vi "Project - Symbols.vi"(7 "Msg Chain":string, 8 "error in (no error)":errorcluster {"code" format="Error %.0f"}, 10 "Project Doc":refnum<class "Project Documentation.lvclass">, 11 "VIDoc Printer - Confluence In":refnum<class "VIDoc Printer - Confluence.lvclass">) -> (0 "error out":errorcluster {"code" format="Error %.0f"}, 3 "VIDoc Printer - Confluence Out":refnum<class "VIDoc Printer - Confluence.lvclass">)   [LabVIEW 2023, in "VIDoc Printer - Confluence.lvlib" / "VIDoc Printer - Confluence.lvclass"]
uses:
  VIDoc Printer - Confluence.lvclass
  Parsing/Project Documentation/Project Documentation.lvclass
  Confluence Formatting/Types/Format Combo Box.ctl
  Parsing/Project Documentation/Project Documentation.lvclass/Project Documentation.ctl
  Parsing/Project Documentation/Get Conditional Disable Symbols.vi
  <userlib>/_PetranWay/LabVIEW Confluence API/Source/Confluence/HTML/Create Table (Responsive).vi
  VIDoc Printer - Confluence.lvclass/VIDoc Printer - Confluence.ctl
  <userlib>/_PetranWay/LabVIEW Confluence API/Source/PetranWay_Confluence API.lvlib
  Confluence Formatting/Confluence Formatting.lvlib
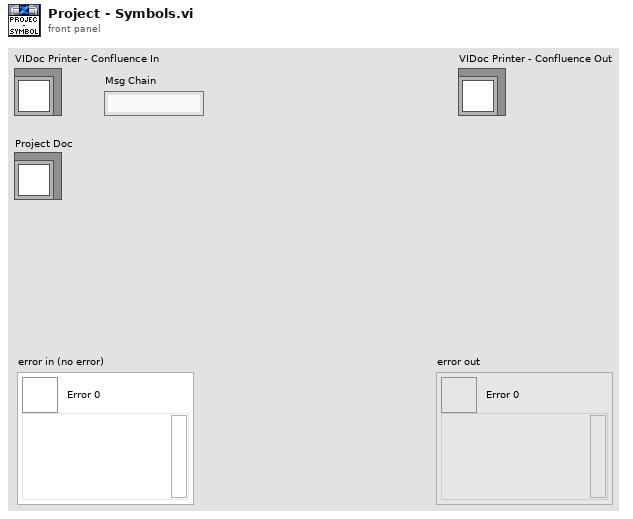
[diagram p1: front panel]
types:
  T1 = typedef "Confluence Formatting.lvlib/Format Combo Box.ctl" = string
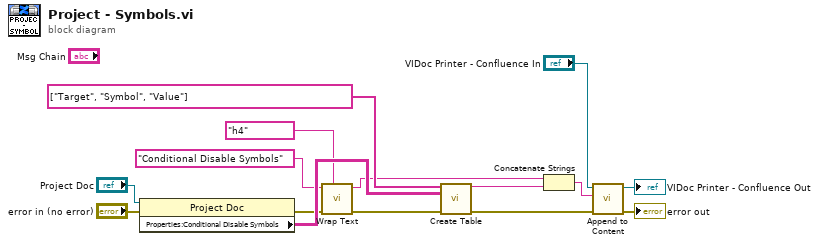
[diagram p0: block diagram]
diagram:
  n1 = property class="Project Doc"(reference="Project Doc", error in="error in (no error)") -> (error out=w6:errorcluster, "Properties:Conditional Disable Symbols"=w9:string[][])  [unwired: 1 out]
  n2 = call "Wrap Text.vi"("Formatting"=T1 "h4", "Error in"=w6, "String"="Conditional Disable Symbols") -> ("Error out"=w5:errorcluster, "Wrapped String"=w3:string)  [unwired: 7 in]
  n3 = call-poly <userlib>:"Create Table.vi"("Headers"=string[] ["Target", "Symbol", "Value"] ("column headers"), "Table Body"=w9, "error in"=w5) -> ("Table HTML"=w1:string, "error out"=w4:errorcluster)  [unwired: 11 in]
  n4 = Concatenate Strings(w3, w1) -> (w2:string)
  n5 = call "Append to Content.vi"("error in (no error)"=w4, "Content"=w2, "VIDoc Printer - Confluence In"="VIDoc Printer - Confluence In") -> ("error out"=→"error out":errorcluster, "VIDoc Printer - Confluence Out"=→"VIDoc Printer - Confluence Out":refnum<class "VIDoc Printer - Confluence.lvclass">)  [unwired: 7 in]
